vi "Handle Message.vi"(7 "priority":T1, 8 "error in (no error)":errorcluster, 10 "Message":refnum<class "Message.lvclass">, 11 "Pub Sub Message Channel in":refnum<class "Pub Sub Message Channel.lvclass">) -> (0 "error out":errorcluster)   [LabVIEW 2020, in "Actor Pub Sub Channels.lvlib" / "Pub Sub Message Channel.lvclass"]
uses:
  Pub Sub Message Channel.lvclass
  <vilib>/ActorFramework/Message Dequeuer/Dequeue Priority.ctl
  <vilib>/ActorFramework/Message/Message.lvclass
  Pub Sub Message Channel.lvclass/Pub Sub Message Channel.ctl
  <vilib>/ActorFramework/Self-Addressed Msg/Self-Addressed Msg.lvclass/Self-Addressed Msg.ctl
  <vilib>/ActorFramework/Message Enqueuer/Message Enqueuer.lvclass
  <vilib>/ActorFramework/Self-Addressed Msg/Self-Addressed Msg.lvclass
  <vilib>/ActorFramework/Message Dequeuer/Message Dequeuer.lvclass
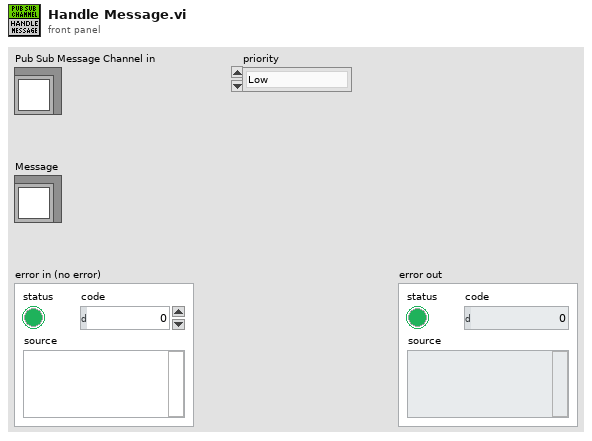
[diagram p1: front panel]
types:
  T1 = typedef "Actor Framework.lvlib/Message Dequeuer.lvclass/Dequeue Priority.ctl" = enum16{"Low", "Normal", "High", "Critical"}
  T2 = map{refnum<class "Message Enqueuer.lvclass">, cluster{"Name":string, "Included (All)":refnum<class "Message.lvclass">[], "Excluded (None)":refnum<class "Message.lvclass">[]}}
  T3 = cluster{"Name":string, "Included (All)":refnum<class "Message.lvclass">[], "Excluded (None)":refnum<class "Message.lvclass">[]}
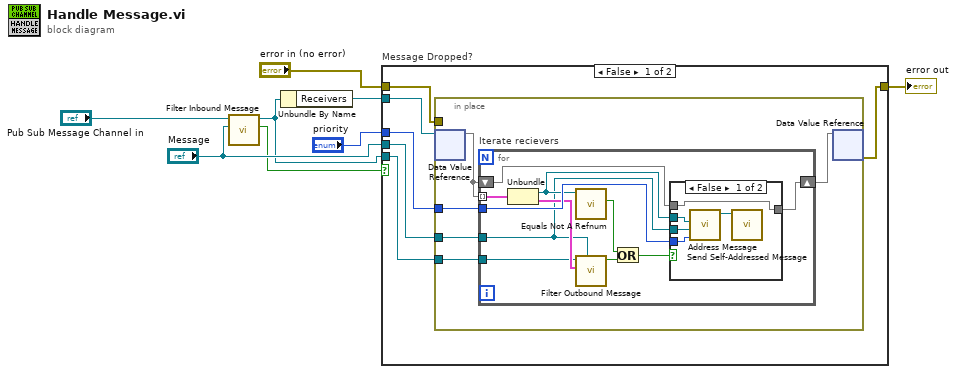
[diagram p0: block diagram]
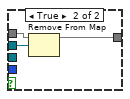
[diagram p2: hidden frame]
diagram:
  n1 = call-dynamic "Filter Inbound Message.vi"("Message"="Message", "Pub Sub Message Channel in"="Pub Sub Message Channel in") -> ("Drop Message"=w2:bool, "Pub Sub Message Channel out"=w1:refnum<class "Pub Sub Message Channel.lvclass">)  [unwired: 8 in]
  n2 = Unbundle By Name(w1) -> ("Receivers"=w6:refnum<data-value>)
  n3 = case "Message Dropped?" shown="False" w2 {
    tunnel: "error in (no error)" -> [w14 w39]
    tunnel: [w13 w39] -> w7
    tunnel: w6 -> [w12 _]
    tunnel: "priority" -> [w11 _]
    tunnel: "Message" -> [w10 _]
    tunnel: w1 -> [w9 _]
    frame False {
      n4 = in-place {
        in-place-border: w10 -> [w19]
        in-place-border: w11 -> [w18]
        in-place-border: w14 -> [_]
        in-place-border: w9 -> [w15]
        n5 = in-place-dvr #1(w12) -> (w17:T2)  [unwired: 1 out]
        n6 = for "Iterate recievers" {
          tunnel: w17 -> [w30] mode=indexing
          tunnel: w19 -> [w21]
          tunnel: w18 -> [w26]
          shift-right: [w28] -> w16
          shift-left: w17 -> [w29]
          tunnel: w15 -> [w22]
          n7 = Unbundle(w30) -> ("Message Enqueuer"=w25:refnum<class "Message Enqueuer.lvclass">, w24:T3)
          n8 = call <vilib>:"Equals Not A Refnum.vi"("Message Enqueuer"=w25) -> ("Not a refnum?"=w27:bool)  [unwired: 10 in]
          n9 = call "Filter Outbound Message.vi"("Message"=w21, "Receiver Info"=w24, "Pub Sub Message Channel in"=w22) -> ("Drop Message"=w20:bool)  [unwired: 8 in]
          n10 = Or(x=w27, y=w20) -> (x .or. y?=w23:bool)
          n11 = case shown="False" w23 {
            tunnel: w29 -> [w31 w38]
            tunnel: [w31 w37] -> w28
            tunnel: w25 -> [w32 w36]
            tunnel: w26 -> [w35 _]
            tunnel: w21 -> [w34 _]
            frame False {
              n12 = call <vilib>:"Address Message.vi"("Message Priority (Normal)"=w35, "Message"=w34, "Destination"=w32) -> ("Self-Addressed Message"=w33:refnum<class "Self-Addressed Msg.lvclass">)  [unwired: 8 in]
              n13 = call-dynamic "Send Self-Addressed Message.vi"("Self-Addressed Message in"=w33) -> ()  [unwired: 9 in, 2 out]
            }
            frame True {
              n14 = Remove From Map(10:w36, 11:w38) -> (3:w37:T2)  [unwired: 2 out]
            }
          }
        }
        n15 = in-place-dvr #1(w16) -> (w13:errorcluster)  [unwired: 1 out]
      }
    }
    frame True {
    }
  }
  "error out" <- w7
